vi "u32 to u8ary.vi"(10 "Numeric":u32 format="%x") -> (2 "Array":u8[](array[numeric]) format="%02x")   [LabVIEW 2019, in "SL_SC.lvlib" / "SL_SC.lvclass"]
uses:
  Library/SL_SC.lvclass
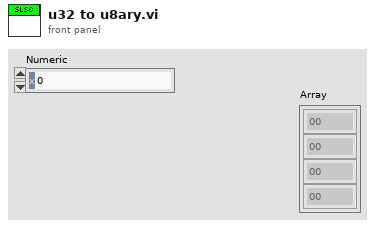
[diagram p1: front panel]
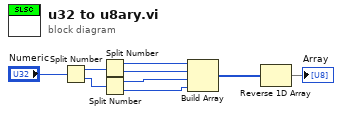
[diagram p0: block diagram]
diagram:
  n1 = Split Number(x="Numeric") -> (hi(x)=w7:u16, lo(x)=w8:u16)
  n2 = Split Number(x=w7) -> (hi(x)=w6:u8, lo(x)=w5:u8)
  n3 = Split Number(x=w8) -> (hi(x)=w4:u8, lo(x)=w3:u8)
  n4 = Build Array(w6, w5, w4, w3) -> (w2:u8[])
  n5 = Reverse 1D Array(array=w2) -> (reversed array=→"Array":u8[])
